vi "AnalysisGUI.Initialize.vi"(8 "error in (no error)":errorcluster, 11 "Refs":T1) -> (0 "error out":errorcluster, 3 "Refs":T1)   [LabVIEW 2015, in "NIAnalysis.lvlib"]
uses:
  NIAnalysis.lvlib
  Types/AnalysisGUI.Refs.ctl
  <vilib>/picture/picture.llb/imagedata.ctl
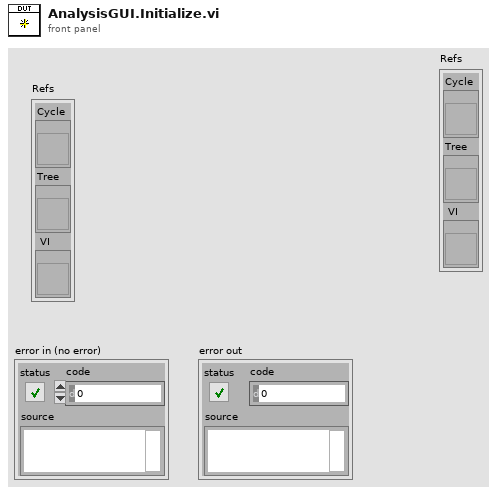
[diagram p1: front panel]
types:
  T1 = typedef "NIAnalysis.lvlib/AnalysisGUI.Refs.ctl" = cluster{"Cycle":refnum<vi>, "Tree":refnum<vi>, " VI":refnum<vi>}
  T2 = typedef "imagedata.ctl" = cluster{"image type":i32, "image depth":i32, "image":u8[], "mask":u8[], "colors":u32[], "Rectangle":cluster{"left":i16, "top":i16, "right":i16, "bottom":i16}}
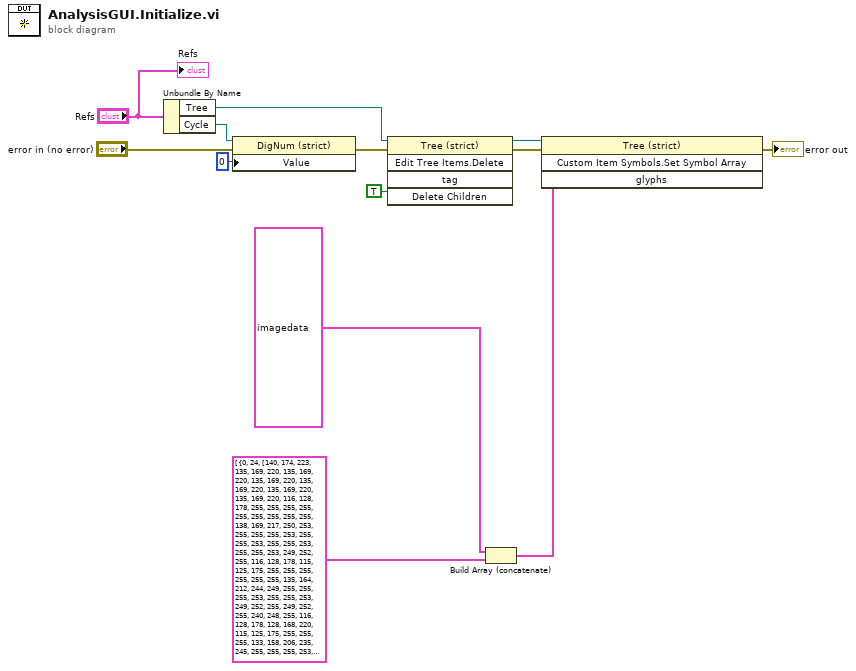
[diagram p0: block diagram]
diagram:
  n1 = Unbundle By Name("Refs") -> ("Tree"=w13:refnum<vi>, "Cycle"=w11:refnum<vi>)
  n2 = property class="DigNum (strict)"(reference=w11, error in="error in (no error)", "Value"=0) -> (error out=w8:errorcluster)  [unwired: 1 out]
  n3 = invoke class="Tree (strict)" method="Edit Tree Items.Delete"(reference=w13, error in=w8, "Delete Children"=TRUE ("Delete Children?")) -> (reference out=w6:refnum<vi>, error out=w5:errorcluster)  [unwired: 2 in, 3 out]
  n4 = Build Array (concatenate)(T2 {"image type"=0, "image depth"=24, "image"=[140, 174, 223, 135, 169, 220, 135, 169, 220, 135, 169, 220, 135, 169, 220, 135, 169, 220, 135, 169, 220, 116, 128, 178, 255, 255, 255, 255, 255, 255, 255, 255, 255, 138, 169, 217, 250, 253, 255, 255, 255, 253, 255, 255, 253, 255, 255, 253, 255, 255, 253, 249, 252, 255, 116, 128, 178, 115, 125, 175, 255, 255, 255, 255, 255, 255, 135, 164, 212, 244, 249, 255, 255, 255, 253, 255, 255, 253, 249, 252, 255, 249, 252, 255, 240, 248, 255, 116, 128, 178, 128, 168, 220, 115, 125, 175, 255, 255, 255, 133, 158, 206, 235, 245, 255, 255, 255, 253, 249, 252, 255, 240, 248, 255, 240, 248, 255, 231, 243, 255, 116, 128, 178, 116, 128, 178, 116, 128, 178, 115, 125, 175, 131, 154, 201, 226, 241, 255, 226, 241, 255, 226, 241, 255, 226, 241, 255, 226, 241, 255, 226, 241, 255, 226, 241, 255, 226, 241, 255, 186, 194, 255, 115, 125, 175, 129, 148, 194, 217, 236, 255, 166, 210, 255, 166, 210, 255, 166, 210, 255, 166, 210, 255, 166, 210, 255, 166, 210, 255, 166, 210, 255, 186, 194, 255, 115, 125, 175, 129, 148, 194, 226, 241, 255, 226, 241, 255, 226, 241, 255, 226, 241, 255, 226, 241, 255, 226, 241, 255, 202, 229, 255, 202, 229, 255, 186, 194, 255, 115, 125, 175, 126, 138, 183, 226, 241, 255, 171, 213, 255, 169, 212, 255, 168, 211, 255, 168, 211, 255, 166, 210, 255, 164, 210, 255, 161, 208, 255, 186, 194, 255, 115, 125, 175, 123, 133, 178, 226, 241, 255, 226, 241, 255, 226, 241, 255, 226, 241, 255, 202, 229, 255, 202, 229, 255, 202, 229, 255, 202, 229, 255, 186, 194, 255, 115, 125, 175, 126, 138, 183, 226, 241, 255, 171, 213, 255, 169, 212, 255, 168, 211, 255, 168, 211, 255, 166, 210, 255, 164, 210, 255, 161, 208, 255, 186, 194, 255, 115, 125, 175, 123, 133, 178, 226, 241, 255, 226, 241, 255, 202, 229, 255, 202, 229, 255, 202, 229, 255, 202, 229, 255, 197, 226, 255, 197, 226, 255, 186, 194, 255, 115, 125, 175, 121, 129, 173, 226, 241, 255, 167, 211, 255, 164, 210, 255, 162, 209, 255, 162, 209, 255, 160, 208, 255, 159, 207, 255, 157, 206, 255, 186, 194, 255, 115, 125, 175, 120, 126, 169, 194, 212, 255, 203, 216, 255, 201, 215, 255, 194, 212, 255, 194, 212, 255, 193, 212, 255, 187, 208, 255, 185, 207, 255, 179, 204, 255, 115, 125, 175, 118, 123, 166, 117, 120, 163, 117, 120, 163, 117, 120, 163, 117, 120, 163, 117, 120, 163, 117, 120, 163, 117, 120, 163, 117, 120, 163, 117, 120, 163, 115, 125, 175], "mask"=[], "colors"=[], "Rectangle"={"left"=0, "top"=0, "right"=11, "bottom"=14}} ("image data"), T2[] [{"image type"=0, "image depth"=24, "image"=[140, 174, 223, 135, 169, 220, 135, 169, 220, 135, 169, 220, 135, 169, 220, 135, 169, 220, 135, 169, 220, 116, 128, 178, 255, 255, 255, 255, 255, 255, 255, 255, 255, 138, 169, 217, 250, 253, 255, 255, 255, 253, 255, 255, 253, 255, 255, 253, 255, 255, 253, 249, 252, 255, 116, 128, 178, 115, 125, 175, 255, 255, 255, 255, 255, 255, 135, 164, 212, 244, 249, 255, 255, 255, 253, 255, 255, 253, 249, 252, 255, 249, 252, 255, 240, 248, 255, 116, 128, 178, 128, 168, 220, 115, 125, 175, 255, 255, 255, 133, 158, 206, 235, 245, 255, 255, 255, 253, 249, 252, 255, 240, 248, 255, 240, 248, 255, 231, 243, 255, 116, 128, 178, 116, 128, 178, 116, 128, 178, 115, 125, 175, 131, 154, 201, 226, 241, 255, 226, 241, 255, 226, 241, 255, 226, 241, 255, 226, 241, 255, 226, 241, 255, 226, 241, 255, 226, 241, 255, 186, 194, 255, 115, 125, 175, 129, 148, 194, 217, 236, 255, 166, 210, 255, 166, 210, 255, 166, 210, 255, 166, 210, 255, 166, 210, 255, 166, 210, 255, 166, 210, 255, 186, 194, 255, 115, 125, 175, 129, 148, 194, 226, 241, 255, 226, 241, 255, 226, 241, 255, 226, 241, 255, 226, 241, 255, 226, 241, 255, 202, 229, 255, 202, 229, 255, 186, 194, 255, 115, 125, 175, 126, 138, 183, 226, 241, 255, 171, 213, 255, 169, 212, 255, 168, 211, 255, 168, 211, 255, 166, 210, 255, 164, 210, 255, 161, 208, 255, 186, 194, 255, 115, 125, 175, 123, 133, 178, 226, 241, 255, 226, 241, 255, 226, 241, 255, 226, 241, 255, 202, 229, 255, 202, 229, 255, 202, 229, 255, 202, 229, 255, 186, 194, 255, 115, 125, 175, 126, 138, 183, 226, 241, 255, 171, 213, 255, 169, 212, 255, 168, 211, 255, 168, 211, 255, 166, 210, 255, 164, 210, 255, 161, 208, 255, 186, 194, 255, 115, 125, 175, 123, 133, 178, 226, 241, 255, 226, 241, 255, 202, 229, 255, 202, 229, 255, 202, 229, 255, 202, 229, 255, 197, 226, 255, 197, 226, 255, 186, 194, 255, 115, 125, 175, 121, 129, 173, 226, 241, 255, 167, 211, 255, 164, 210, 255, 162, 209, 255, 162, 209, 255, 160, 208, 255, 159, 207, 255, 157, 206, 255, 186, 194, 255, 115, 125, 175, 120, 126, 169, 194, 212, 255, 203, 216, 255, 201, 215, 255, 194, 212, 255, 194, 212, 255, 193, 212, 255, 187, 208, 255, 185, 207, 255, 179, 204, 255, 115, 125, 175, 118, 123, 166, 117, 120, 163, 117, 120, 163, 117, 120, 163, 117, 120, 163, 117, 120, 163, 117, 120, 163, 117, 120, 163, 117, 120, 163, 117, 120, 163, 115, 125, 175], "mask"=[], "colors"=[], "Rectangle"={"left"=0, "top"=0, "right"=11, "bottom"=14}}, {"image type"=0, "image depth"=32, "image"=[0, 255, 255, 255, 0, 255, 255, 255, 0, 255, 255, 255, 0, 255, 255, 255, 0, 255, 255, 255, 0, 255, 255, 255, 0, 255, 255, 255, 0, 255, 255, 255, 0, 255, 255, 255, 0, 255, 255, 255, 0, 255, 255, 255, 0, 255, 255, 255, 0, 255, 255, 255, 0, 255, 255, 255, 0, 255, 255, 255, 0, 255, 255, 255, 255, 71, 125, 180, 255, 71, 125, 180, 255, 71, 125, 180, 0, 255, 255, 255, 0, 255, 255, 255, 0, 255, 255, 255, 0, 255, 255, 255, 0, 255, 255, 255, 0, 255, 255, 255, 0, 255, 255, 255, 0, 255, 255, 255, 0, 255, 255, 255, 0, 255, 255, 255, 0, 255, 255, 255, 0, 255, 255, 255, 0, 255, 255, 255, 255, 71, 125, 180, 255, 253, 253, 253, 255, 253, 253, 253, 0, 255, 255, 255, 0, 255, 255, 255, 0, 255, 255, 255, 0, 255, 255, 255, 0, 255, 255, 255, 0, 255, 255, 255, 0, 255, 255, 255, 0, 255, 255, 255, 0, 255, 255, 255, 0, 255, 255, 255, 0, 255, 255, 255, 0, 255, 255, 255, 0, 255, 255, 255, 255, 71, 125, 180, 255, 253, 253, 253, 255, 71, 125, 180, 0, 255, 255, 255, 0, 255, 255, 255, 0, 255, 255, 255, 0, 255, 255, 255, 0, 255, 255, 255, 0, 255, 255, 255, 0, 255, 255, 255, 0, 255, 255, 255, 0, 255, 255, 255, 0, 255, 255, 255, 0, 255, 255, 255, 0, 255, 255, 255, 0, 255, 255, 255, 255, 71, 125, 180, 255, 253, 253, 253, 255, 253, 253, 253, 0, 255, 255, 255, 255, 71, 125, 180, 255, 71, 125, 180, 255, 71, 125, 180, 0, 255, 255, 255, 0, 255, 255, 255, 0, 255, 255, 255, 0, 255, 255, 255, 0, 255, 255, 255, 0, 255, 255, 255, 0, 255, 255, 255, 0, 255, 255, 255, 0, 255, 255, 255, 255, 71, 125, 180, 255, 253, 253, 253, 255, 71, 125, 180, 0, 255, 255, 255, 255, 71, 125, 180, 255, 253, 253, 253, 255, 253, 253, 253, 0, 255, 255, 255, 0, 255, 255, 255, 0, 255, 255, 255, 0, 255, 255, 255, 0, 255, 255, 255, 0, 255, 255, 255, 0, 255, 255, 255, 0, 255, 255, 255, 0, 255, 255, 255, 255, 71, 125, 180, 255, 253, 253, 253, 255, 253, 253, 253, 0, 255, 255, 255, 255, 71, 125, 180, 255, 253, 253, 253, 255, 71, 125, 180, 0, 255, 255, 255, 0, 255, 255, 255, 0, 255, 255, 255, 0, 255, 255, 255, 0, 255, 255, 255, 0, 255, 255, 255, 0, 255, 255, 255, 0, 255, 255, 255, 0, 255, 255, 255, 255, 71, 125, 180, 255, 253, 253, 253, 255, 71, 125, 180, 0, 255, 255, 255, 255, 71, 125, 180, 255, 253, 253, 253, 255, 253, 253, 253, 0, 255, 255, 255, 255, 71, 125, 180, 255, 71, 125, 180, 255, 71, 125, 180, 0, 255, 255, 255, 0, 255, 255, 255, 0, 255, 255, 255, 0, 255, 255, 255, 0, 255, 255, 255, 255, 71, 125, 180, 255, 253, 253, 253, 255, 253, 253, 253, 0, 255, 255, 255, 255, 71, 125, 180, 255, 253, 253, 253, 255, 71, 125, 180, 0, 255, 255, 255, 255, 71, 125, 180, 255, 253, 253, 253, 255, 253, 253, 253, 0, 255, 255, 255, 0, 255, 255, 255, 0, 255, 255, 255, 0, 255, 255, 255, 0, 255, 255, 255, 255, 71, 125, 180, 255, 253, 253, 253, 255, 71, 125, 180, 0, 255, 255, 255, 255, 71, 125, 180, 255, 253, 253, 253, 255, 253, 253, 253, 0, 255, 255, 255, 255, 71, 125, 180, 255, 253, 253, 253, 255, 71, 125, 180, 0, 255, 255, 255, 0, 255, 255, 255, 0, 255, 255, 255, 0, 255, 255, 255, 0, 255, 255, 255, 255, 71, 125, 180, 255, 253, 253, 253, 255, 253, 253, 253, 0, 255, 255, 255, 255, 71, 125, 180, 255, 253, 253, 253, 255, 71, 125, 180, 0, 255, 255, 255, 255, 71, 125, 180, 255, 253, 253, 253, 255, 253, 253, 253, 0, 255, 255, 255, 255, 71, 125, 180, 255, 71, 125, 180, 255, 71, 125, 180, 0, 255, 255, 255, 255, 71, 125, 180, 255, 253, 253, 253, 255, 71, 125, 180, 0, 255, 255, 255, 255, 71, 125, 180, 255, 253, 253, 253, 255, 253, 253, 253, 0, 255, 255, 255, 255, 71, 125, 180, 255, 253, 253, 253, 255, 71, 125, 180, 0, 255, 255, 255, 255, 71, 125, 180, 255, 253, 253, 253, 255, 253, 253, 253, 0, 255, 255, 255, 255, 71, 125, 180, 255, 253, 253, 253, 255, 253, 253, 253, 0, 255, 255, 255, 255, 71, 125, 180, 255, 253, 253, 253, 255, 71, 125, 180, 0, 255, 255, 255, 255, 71, 125, 180, 255, 253, 253, 253, 255, 253, 253, 253, 0, 255, 255, 255, 255, 71, 125, 180, 255, 253, 253, 253, 255, 71, 125, 180, 0, 255, 255, 255, 255, 71, 125, 180, 255, 253, 253, 253, 255, 71, 125, 180, 0, 255, 255, 255, 255, 71, 125, 180, 255, 253, 253, 253, 255, 253, 253, 253, 0, 255, 255, 255, 255, 71, 125, 180, 255, 253, 253, 253, 255, 71, 125, 180, 0, 255, 255, 255, 255, 71, 125, 180, 255, 253, 253, 253, 255, 253, 253, 253, 0, 255, 255, 255, 255, 71, 125, 180, 255, 253, 253, 253, 255, 253, 253, 253, 0, 255, 255, 255, 255, 71, 125, 180, 255, 253, 253, 253, 255, 71, 125, 180, 0, 255, 255, 255, 255, 71, 125, 180, 255, 253, 253, 253, 255, 253, 253, 253, 0, 255, 255, 255, 255, 71, 125, 180, 255, 253, 253, 253, 255, 71, 125, 180, 0, 255, 255, 255, 0, 255, 255, 255, 0, 255, 255, 255, 0, 255, 255, 255, 0, 255, 255, 255, 0, 255, 255, 255, 0, 255, 255, 255, 0, 255, 255, 255, 0, 255, 255, 255, 0, 255, 255, 255, 0, 255, 255, 255, 0, 255, 255, 255, 0, 255, 255, 255, 0, 255, 255, 255, 0, 255, 255, 255, 0, 255, 255, 255, 0, 255, 255, 255], "mask"=[0, 0, 224, 0, 224, 0, 224, 0, 238, 0, 238, 0, 238, 0, 238, 224, 238, 224, 238, 224, 238, 238, 238, 238, 238, 238, 238, 238, 238, 238, 0, 0], "colors"=[], "Rectangle"={"left"=0, "top"=0, "right"=16, "bottom"=16}}, {"image type"=0, "image depth"=32, "image"=[255, 255, 255, 255, 255, 255, 255, 255, 255, 255, 255, 255, 255, 255, 255, 255, 255, 255, 255, 255, 255, 255, 255, 255, 255, 255, 255, 255, 255, 255, 255, 255, 255, 255, 255, 255, 255, 255, 255, 255, 255, 255, 255, 255, 255, 255, 255, 255, 255, 255, 255, 255, 255, 255, 255, 255, 255, 255, 255, 255, 255, 255, 255, 255, 255, 255, 255, 255, 255, 255, 255, 255, 255, 255, 255, 255, 255, 255, 255, 255, 255, 255, 255, 255, 255, 255, 255, 255, 255, 255, 255, 255, 255, 255, 255, 255, 255, 255, 255, 255, 255, 255, 255, 255, 255, 255, 255, 255, 255, 255, 255, 255, 255, 255, 255, 255, 255, 255, 255, 255, 255, 255, 255, 255, 255, 255, 255, 255, 255, 255, 255, 255, 255, 255, 255, 255, 255, 255, 255, 255, 255, 255, 255, 255, 255, 255, 255, 255, 255, 255, 255, 255, 255, 255, 0, 0, 255, 255, 255, 255, 255, 255, 255, 255, 255, 255, 255, 255, 255, 255, 255, 255, 255, 255, 255, 255, 255, 255, 255, 255, 255, 255, 255, 255, 255, 255, 255, 255, 255, 255, 255, 255, 255, 255, 255, 255, 255, 255, 255, 255, 255, 255, 255, 255, 255, 255, 255, 255, 255, 255, 255, 255, 255, 255, 0, 0, 255, 255, 255, 255, 255, 255, 0, 0, 255, 255, 255, 255, 255, 255, 255, 255, 255, 255, 255, 255, 255, 255, 255, 255, 255, 255, 255, 255, 255, 255, 255, 255, 255, 255, 0, 0, 255, 255, 255, 255, 255, 255, 255, 255, 255, 255, 0, 0, 255, 255, 0, 0, 255, 255, 0, 0, 255, 255, 255, 255, 255, 255, 0, 0, 255, 255, 255, 255, 255, 255, 0, 0, 255, 255, 255, 255, 255, 255, 255, 255, 255, 255, 255, 255, 255, 255, 255, 255, 255, 255, 255, 255, 255, 255, 0, 0, 255, 255, 255, 255, 255, 255, 0, 0, 255, 255, 255, 255, 255, 255, 0, 0, 255, 255, 255, 255, 255, 255, 0, 0, 255, 255, 255, 255, 255, 255, 0, 0, 255, 255, 255, 255, 255, 255, 0, 0, 255, 255, 255, 255, 255, 255, 255, 255, 255, 255, 255, 255, 255, 255, 255, 255, 255, 255, 255, 255, 255, 255, 0, 0, 255, 255, 255, 255, 255, 255, 0, 0, 255, 255, 255, 255, 255, 255, 0, 0, 255, 255, 255, 255, 255, 255, 0, 0, 255, 255, 255, 255, 255, 255, 0, 0, 255, 255, 255, 255, 255, 255, 0, 0, 255, 255, 255, 255, 255, 255, 0, 0, 255, 255, 0, 0, 255, 255, 0, 0, 255, 255, 255, 255, 255, 255, 0, 0, 255, 255, 255, 255, 255, 255, 0, 0, 255, 255, 255, 255, 255, 255, 0, 0, 255, 255, 255, 255, 255, 255, 0, 0, 255, 255, 255, 255, 255, 255, 0, 0, 255, 255, 255, 255, 255, 255, 0, 0, 255, 255, 255, 255, 255, 255, 0, 0, 255, 255, 255, 255, 255, 255, 0, 0, 255, 255, 255, 255, 255, 255, 0, 0, 255, 255, 255, 255, 255, 255, 0, 0, 255, 255, 0, 0, 255, 255, 255, 255, 255, 255, 255, 255, 255, 255, 0, 0, 255, 255, 0, 0, 255, 255, 0, 0, 255, 255, 255, 255, 255, 255, 0, 0, 255, 255, 255, 255, 255, 255, 0, 0, 255, 255, 255, 255, 255, 255, 0, 0, 255, 255, 255, 255, 255, 255, 0, 0, 255, 255, 255, 255, 255, 255, 0, 0, 255, 255, 255, 255, 255, 255, 255, 255, 255, 255, 255, 255, 255, 255, 255, 255, 255, 255, 255, 255, 255, 255, 255, 255, 255, 255, 255, 255, 255, 255, 0, 0, 255, 255, 255, 255, 255, 255, 0, 0, 255, 255, 255, 255, 255, 255, 0, 0, 255, 255, 0, 0, 255, 255, 0, 0, 255, 255, 255, 255, 255, 255, 0, 0, 255, 255, 255, 255, 255, 255, 255, 255, 255, 255, 255, 255, 255, 255, 255, 255, 255, 255, 255, 255, 255, 255, 255, 255, 255, 255, 255, 255, 255, 255, 0, 0, 255, 255, 255, 255, 255, 255, 0, 0, 255, 255, 255, 255, 255, 255, 255, 255, 255, 255, 255, 255, 255, 255, 255, 255, 255, 255, 255, 255, 255, 255, 0, 0, 255, 255, 255, 255, 255, 255, 255, 255, 255, 255, 255, 255, 255, 255, 255, 255, 255, 255, 255, 255, 255, 255, 255, 255, 255, 255, 255, 255, 255, 255, 255, 255, 255, 255, 0, 0, 255, 255, 255, 255, 255, 255, 255, 255, 255, 255, 255, 255, 255, 255, 255, 255, 255, 255, 255, 255, 255, 255, 255, 255, 255, 255, 0, 0, 255, 255, 255, 255, 255, 255, 255, 255, 255, 255, 255, 255, 255, 255, 255, 255, 255, 255, 255, 255, 255, 255, 255, 255, 255, 255, 255, 255, 255, 255, 255, 255, 255, 255, 255, 255, 255, 255, 255, 255, 255, 255, 255, 255, 255, 255, 255, 255, 255, 255, 255, 255, 255, 255, 255, 255, 255, 255, 255, 255, 255, 255, 255, 255], "mask"=[255, 255, 255, 255, 255, 255, 255, 255, 255, 255, 255, 255, 255, 255, 255, 255, 255, 255, 255, 255, 255, 255, 255, 255, 255, 255], "colors"=[], "Rectangle"={"left"=0, "top"=0, "right"=16, "bottom"=13}}, {"image type"=0, "image depth"=24, "image"=[153, 153, 153, 153, 153, 153, 153, 153, 153, 153, 153, 153, 153, 153, 153, 153, 153, 153, 153, 153, 153, 153, 153, 153, 153, 153, 153, 153, 153, 153, 153, 153, 153, 153, 153, 153, 153, 153, 153, 153, 153, 153, 153, 153, 153, 153, 153, 153, 0, 0, 0, 0, 0, 0, 0, 0, 0, 0, 0, 0, 0, 0, 0, 0, 0, 0, 0, 0, 0, 0, 0, 0, 0, 0, 0, 0, 0, 0, 0, 0, 0, 0, 0, 0, 0, 0, 0, 0, 0, 0, 0, 0, 0, 0, 0, 0, 0, 0, 0, 255, 255, 0, 255, 255, 0, 255, 255, 0, 255, 255, 0, 255, 255, 0, 255, 255, 0, 255, 255, 0, 255, 255, 0, 255, 255, 0, 255, 255, 0, 255, 255, 0, 255, 255, 0, 255, 255, 0, 255, 255, 0, 255, 255, 0, 0, 0, 0, 255, 255, 0, 0, 0, 0, 255, 255, 0, 255, 255, 0, 255, 255, 0, 0, 0, 0, 255, 255, 0, 255, 255, 0, 255, 255, 0, 0, 0, 0, 255, 255, 0, 255, 255, 0, 255, 255, 0, 0, 0, 0, 255, 255, 0, 0, 0, 0, 255, 255, 0, 0, 0, 0, 255, 255, 0, 0, 0, 0, 255, 255, 0, 0, 0, 0, 255, 255, 0, 0, 0, 0, 255, 255, 0, 0, 0, 0, 255, 255, 0, 0, 0, 0, 255, 255, 0, 0, 0, 0, 255, 255, 0, 0, 0, 0, 0, 0, 0, 0, 0, 0, 0, 0, 0, 0, 0, 0, 0, 0, 0, 0, 0, 0, 0, 0, 0, 0, 0, 0, 0, 0, 0, 0, 0, 0, 0, 0, 0, 0, 0, 0, 0, 0, 0, 0, 0, 0, 0, 0, 0], "mask"=[], "colors"=[], "Rectangle"={"left"=0, "top"=0, "right"=16, "bottom"=6}}, {"image type"=0, "image depth"=24, "image"=[0, 0, 0, 0, 0, 0, 0, 0, 0, 0, 0, 0, 0, 0, 0, 0, 0, 0, 0, 0, 0, 0, 0, 0, 0, 0, 0, 0, 0, 0, 0, 0, 0, 0, 0, 0, 0, 0, 0, 0, 0, 0, 255, 255, 255, 0, 0, 0, 255, 255, 211, 255, 255, 211, 255, 255, 211, 255, 255, 211, 255, 255, 211, 255, 255, 211, 255, 255, 211, 255, 255, 211, 255, 255, 211, 255, 255, 211, 255, 255, 211, 255, 255, 211, 0, 0, 0, 128, 128, 128, 0, 0, 0, 255, 255, 211, 255, 255, 211, 255, 255, 211, 255, 255, 211, 255, 255, 211, 255, 255, 211, 255, 255, 211, 0, 0, 0, 0, 0, 0, 255, 255, 211, 255, 255, 211, 255, 255, 211, 0, 0, 0, 128, 128, 128, 0, 0, 0, 255, 255, 211, 255, 255, 211, 255, 255, 211, 255, 255, 211, 255, 255, 211, 255, 255, 211, 0, 0, 0, 0, 0, 0, 0, 0, 0, 0, 0, 0, 255, 255, 211, 255, 255, 211, 0, 0, 0, 128, 128, 128, 0, 0, 0, 255, 255, 211, 255, 255, 211, 0, 0, 0, 0, 0, 0, 0, 0, 0, 0, 0, 0, 0, 0, 0, 0, 0, 0, 255, 255, 211, 255, 255, 211, 255, 255, 211, 255, 255, 211, 0, 0, 0, 128, 128, 128, 0, 0, 0, 255, 255, 211, 255, 255, 211, 0, 0, 0, 0, 0, 0, 0, 0, 0, 0, 0, 0, 0, 0, 0, 0, 0, 0, 255, 255, 211, 255, 255, 211, 255, 255, 211, 255, 255, 211, 0, 0, 0, 128, 128, 128, 0, 0, 0, 255, 255, 211, 255, 255, 211, 255, 255, 211, 255, 255, 211, 255, 255, 211, 255, 255, 211, 0, 0, 0, 0, 0, 0, 0, 0, 0, 0, 0, 0, 255, 255, 211, 255, 255, 211, 0, 0, 0, 128, 128, 128, 0, 0, 0, 255, 255, 211, 255, 255, 211, 255, 255, 211, 255, 255, 211, 255, 255, 211, 255, 255, 211, 255, 255, 211, 0, 0, 0, 0, 0, 0, 255, 255, 211, 255, 255, 211, 255, 255, 211, 0, 0, 0, 128, 128, 128, 0, 0, 0, 255, 255, 211, 255, 255, 211, 255, 255, 211, 255, 255, 211, 255, 255, 211, 255, 255, 211, 255, 255, 211, 255, 255, 211, 255, 255, 211, 255, 255, 211, 255, 255, 211, 255, 255, 211, 0, 0, 0, 128, 128, 128, 0, 0, 0, 0, 0, 0, 0, 0, 0, 0, 0, 0, 0, 0, 0, 0, 0, 0, 0, 0, 0, 0, 0, 0, 0, 0, 0, 0, 0, 0, 0, 0, 0, 0, 0, 0, 0, 0, 0, 0, 0, 0, 128, 128, 128, 255, 255, 255, 128, 128, 128, 128, 128, 128, 128, 128, 128, 128, 128, 128, 128, 128, 128, 128, 128, 128, 128, 128, 128, 128, 128, 128, 128, 128, 128, 128, 128, 128, 128, 128, 128, 128, 128, 128, 128, 128, 128, 128, 128, 128], "mask"=[], "colors"=[], "Rectangle"={"left"=0, "top"=0, "right"=15, "bottom"=11}}] ("Array")) -> (w1:T2[])
  n5 = invoke class="Tree (strict)" method="Custom Item Symbols.Set Symbol Array"(reference=w6, error in=w5, "glyphs"=w1) -> (error out=→"error out":errorcluster)  [unwired: 1 in, 3 out]
  "Refs" <- "Refs"
